vi "EMV Slope Flow Detector.vi"(8 "error in (no error)":errorcluster, 11 "Current T6 Temperatures in":dbl[](array[numeric])) -> (0 "error out":errorcluster, 1 "slope":dbl, 2 "standard deviation":dbl format="%0.2f", 3 "Current T6 Temperatures out":dbl[](array[numeric]), 5 "mean":dbl format="%0.2f")   [LabVIEW 2016]
uses:
  <vilib>/Analysis/6fits.llb/Curve Fitting Criteria.ctl
  <vilib>/Analysis/NI_AALPro.lvlib
  <vilib>/Analysis/NI_AALBase.lvlib
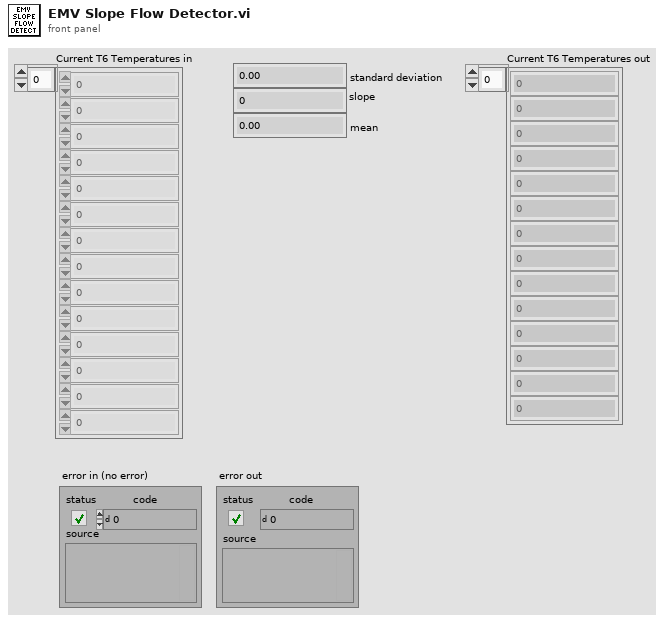
[diagram p1: front panel]
types:
  T1 = typedef "NI_AALPro.lvlib/Curve Fitting Criteria.ctl" = u16
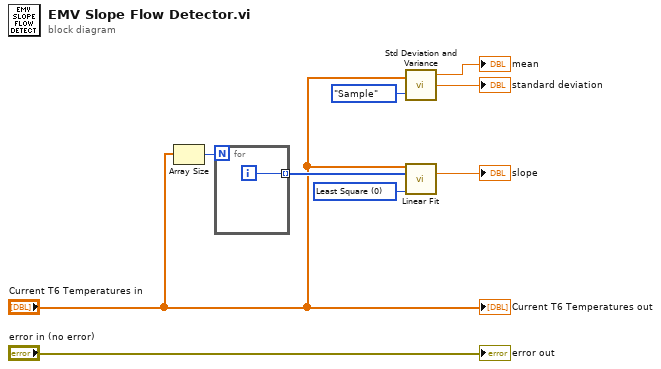
[diagram p0: block diagram]
diagram:
  w7 = T1 0 items=["Least Square", "Least Absolute Residual", "Bisquare"] ("method")
  n1 = Array Size(array="Current T6 Temperatures in") -> (size(s)=w4:i32)
  n2 = for {
    N: w4 -> [_]
    tunnel: [w10] -> w5 mode=indexing
    i -> [w10]
  }
  n3 = call <vilib>:"Std Deviation and Variance.vi"("X"="Current T6 Temperatures in", "Weighting (Sample)"=enum16{"Sample", "Population"}."Sample") -> ("mean"=→"mean":dbl, "standard deviation"=→"standard deviation":dbl)  [unwired: 1 out]
  n4 = call <vilib>:"Linear Fit.vi"("Y"="Current T6 Temperatures in", "X"=w5, "method"=w7) -> ("slope"=→"slope":dbl)  [unwired: 8 in, 4 out]
  "error out" <- "error in (no error)"
  "Current T6 Temperatures out" <- "Current T6 Temperatures in"
